vi "Hold.vi"(8 "error in (no error)":errorcluster, 11 "Instrument.1820 in":refnum<class "Instrument.Oxford1820.lvclass">) -> (0 "error out":errorcluster, 2 "Response":string, 3 "Instrument.1820 in":refnum<class "Instrument.Oxford1820.lvclass">)   [LabVIEW 2019, in "Instrument.Oxford1820.lvclass"]
uses:
  Instrument.Oxford1820.lvclass
  Typedefs/Instrument.Oxford1820.protectedCommands-enum.ctl
  0c1d408f-5749-481e-8a9e-104c5a6b3b94.vi/c1212cb4-0bc1-4061-891e-76a5034669e6.vi
  0c1d408f-5749-481e-8a9e-104c5a6b3b94.vi/6f7a4645-c0c1-45d5-b490-09ceb1147cea.vi
  <vilib>/Utility/Data Type/Get Type Information.vi
  <vilib>/JDP Science/JSONtext/JSON text to Variant.vi
  <vilib>/JDP Science/JSONtext/LVClass Serializer/JSONtext LVClass Serializer.lvclass
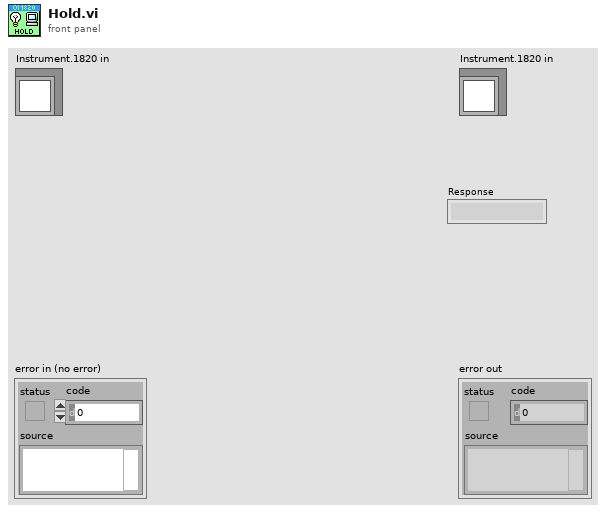
[diagram p1: front panel]
types:
  T1 = typedef "Instrument.Oxford1820.lvclass/Instrument.Oxford1820.protectedCommands-enum.ctl" = enum16{"Hold", "RampToSet", "RampToZero", "Clamp", "setTarget", "setSwitchHeat", "setLambda", "setFillMode", "setNeedleValve", "getStatus", "getTarget", "getSwitchHeat", "getPSUField", "setSequenceStatus"}
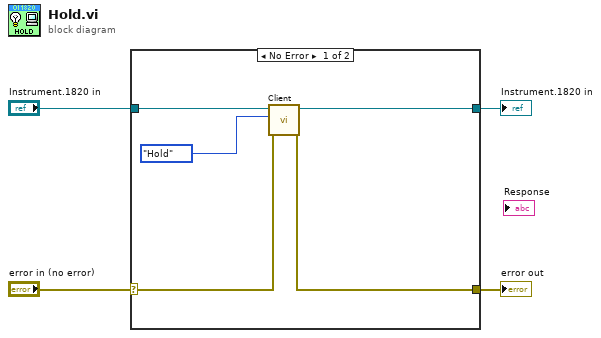
[diagram p0: block diagram]
diagram:
  n1 = case shown="No Error" "error in (no error)" {
    selector: "error in (no error)" -> [w7 w11]
    tunnel: [w5 w11] -> w3
    tunnel: [w8 w10] -> w1
    tunnel: "Instrument.1820 in" -> [w9 w10]
    frame No Error {
      n2 = call-dynamic "Client.vi"("error in (no error)"=w7, "Command in"=Instrument.Oxford1820.protectedCommands-enum."Hold" ("protectedCommands"), "Instrument in"=w9) -> ("error out"=w5:errorcluster, "Instrument out"=w8:refnum<class "Instrument.Oxford1820.lvclass">)  [unwired: 5 in, 2 out]
    }
    frame Error {
    }
  }
  "error out" <- w3
  "Instrument.1820 in" <- w1
